vi "cal_max_min_y.vi"(10 "Position 2":cluster{"Left":i32, "Top":i32}, 11 "Position 1":cluster{"Left":i32, "Top":i32}) -> (2 "min y":i32, 3 "max y":i32)   [LabVIEW 2018]
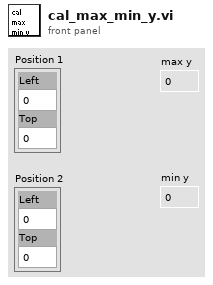
[diagram p1: front panel]
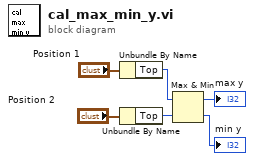
[diagram p0: block diagram]
diagram:
  n1 = Unbundle By Name("Position 1") -> ("Top"=w2:i32)
  n2 = Unbundle By Name("Position 2") -> ("Top"=w3:i32)
  n3 = Max & Min(x=w2, y=w3) -> (max(x,y)=→"max y":i32, min(x,y)=→"min y":i32)
